vi "Add Files to Project (SubVI).vi"(8 "error out 2":errorcluster, 10 "Custom Device Library":path, 11 "Custom Device Folder":path) -> ()   [LabVIEW 2010]
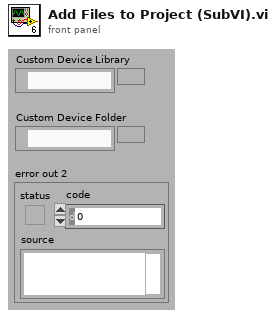
[diagram p1: front panel]
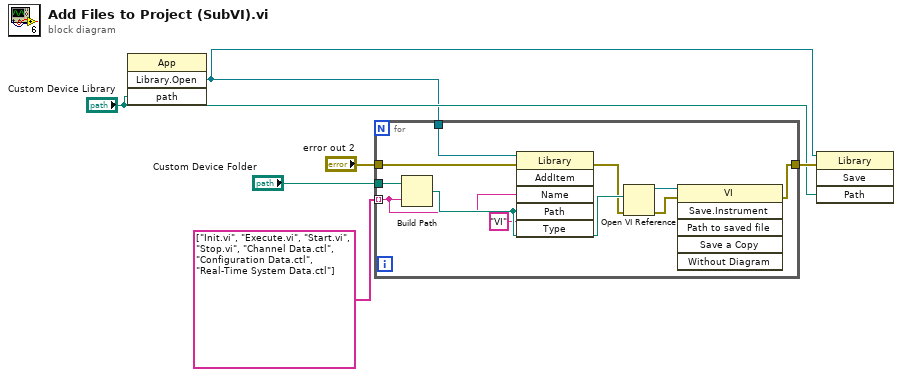
[diagram p0: block diagram]
diagram:
  n1 = invoke class="App" method="Library.Open"("path"="Custom Device Library") -> ("Open Library"=w1:refnum<vi>)  [unwired: 3 in, 3 out]
  n2 = for {
    tunnel: "Custom Device Folder" -> [w16]
    tunnel: string[] ["Init.vi", "Execute.vi", "Start.vi", "Stop.vi", "Channel Data.ctl", "Configuration Data.ctl", "Real-Time System Data.ctl"] -> [w8] mode=indexing
    tunnel: "error out 2" -> [w15]
    tunnel: [w9] -> w6
    tunnel: w1 -> [w14]
    n3 = Build Path(base path=w16, name or relative path=w8) -> (appended path=w11:path)
    n4 = invoke class="Library" method="AddItem"(reference=w14, error in=w15, "Name"=w8, "Path"=w11, "Type"="VI") -> (error out=w10:errorcluster)  [unwired: 1 in, 5 out]
    n5 = Open VI Reference(vi path=w11, error in (no error)=w10) -> (vi reference=w12:refnum<vi>, error out=w13:errorcluster)  [unwired: 4 in]
    n6 = invoke class="VI" method="Save.Instrument"(reference=w12, error in=w13) -> (error out=w9:errorcluster)  [unwired: 4 in, 5 out]
  }
  n7 = invoke class="Library" method="Save"(reference=w1, error in=w6, "Path"="Custom Device Library") -> ()  [unwired: 1 in, 4 out]
